vi "SLSC_Check Connection and Module.vi"(6 "Connect timeout (s)":dbl=4.0 format="%#_13g", 8 "error in (no error)":errorcluster, 10 "Supported Modules":T1[](array[typedef]), 11 "devices":refnum<k21>) -> (0 "error out":errorcluster, 3 "Device Found?":bool)   [LabVIEW 2015, in "SLSC CD Engine.lvlib"]
uses:
  SLSC CD API/SLSC CD Engine/SLSC CD Engine.lvlib
  SLSC CD API/SLSC CD Engine/SLSC Identification.ctl
  <vilib>/SLSC/Initialize Session with Devices.vi
  <vilib>/SLSC/Close Session.vi
  <vilib>/SLSC/SLSC.lvlib
  <resource>/objmgr/slsc.rc
  SLSC CD API/SLSC CD Shared/SLSC CD Shared.lvlib
panel:
  out "Supported Modules":T2(array[cluster]) {"Dev.ProductNumber" format="%.0x"; "Dev.VendorNumber" format="%.0x"}
  out "Dev.VendorNum":u32 format="%.0x"
  out "Dev.ProductNum":u32 format="%.0x"
  out "Dev.ProductName":string
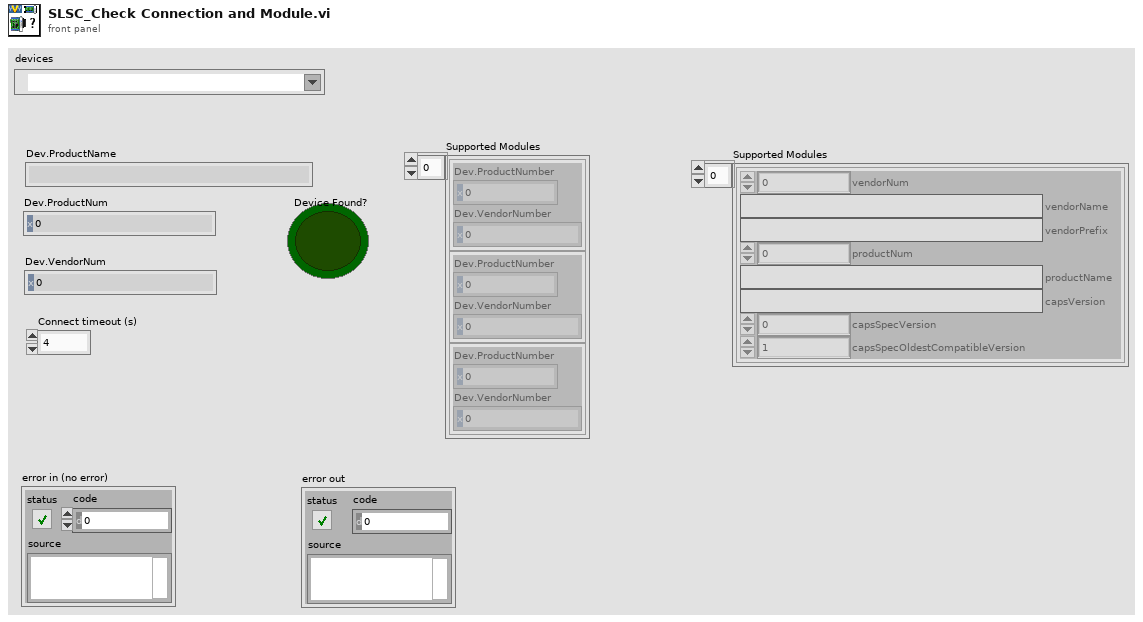
[diagram p1: front panel]
types:
  T1 = typedef "SLSC CD Shared.lvlib/SLSC Identification.ctl" = cluster{"vendorName":string, "productNum":u32, "capsVersion":string, "capsSpecVersion":u32, "productName":string, "vendorNum":u32, "vendorPrefix":string, "capsSpecOldestCompatibleVersion":u32}
  T2 = cluster{"Dev.ProductNumber":u32, "Dev.VendorNumber":u32}[]
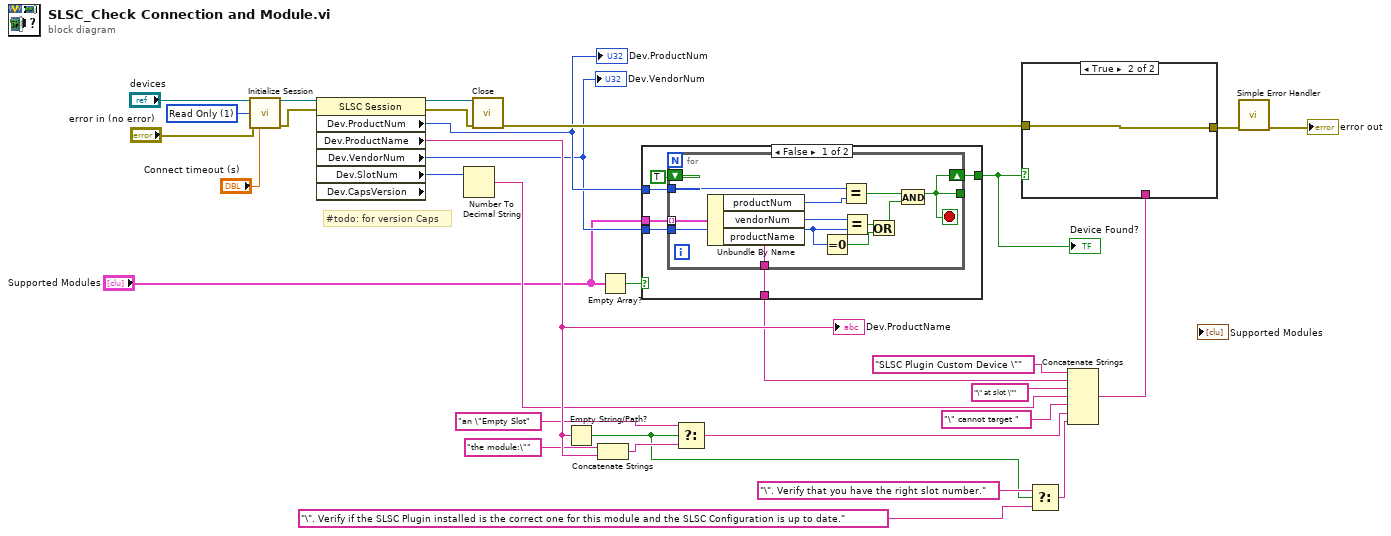
[diagram p0: block diagram]
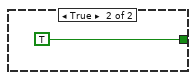
[diagram p2: hidden frame]
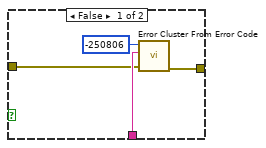
[diagram p3: hidden frame]
diagram:
  w8 = 1 items=["None"=0, "Read Only"=1, "Read/Write"=3] ("reservation access (Read/Write)")
  # "#todo: for version Caps"
  n1 = call-poly <vilib>:"Initialize Session.vi"("devices"="devices", "reservation access (Read/Write)"=w8, "error in (no error)"="error in (no error)", "connect timeout (60 sec)"="Connect timeout (s)") -> ("session out"=w13:refnum<k21>, "error out"=w12:errorcluster)  [unwired: 10 in]
  n2 = property class="SLSC Session" props=["Dev.ProductNum", "Dev.ProductName", "Dev.VendorNum", "Dev.SlotNum", "Dev.CapsVersion"](reference=w13, error in=w12) -> (reference out=w11:refnum<k21>, error out=w10:errorcluster, "Dev.ProductNum"=w18:u32, "Dev.ProductName"=w27:string, "Dev.VendorNum"=w17:u32, "Dev.SlotNum"=w7:u32)  [unwired: 1 out]
  "Dev.ProductName" <- w27
  "Dev.ProductNum" <- w18
  "Dev.VendorNum" <- w17
  n3 = Number To Decimal String(number=w7) -> (decimal integer string=w14:string)  [unwired: 1 in]
  n4 = call-poly <vilib>:"Close.vi"("session in"=w11, "error in (no error)"=w10) -> ("error out"=w32:errorcluster)  [unwired: 13 in]
  n5 = Empty String/Path?(string/path=w27) -> (empty?=w19:bool)
  n6 = Concatenate Strings("the module:\"" ("error message (\"\")"), w27) -> (w25:string)
  n7 = Empty Array?(array="Supported Modules") -> (empty?=w9:bool)
  n8 = case shown="False" w9 {
    tunnel: w18 -> [w37 _]
    tunnel: "Supported Modules" -> [w36 _]
    tunnel: w17 -> [w35 _]
    tunnel: [w34 TRUE] -> w1
    tunnel: [w33 _] -> w2
    frame False {
      n9 = for {
        tunnel: w37 -> [w49]
        tunnel: w36 -> [w40] mode=indexing
        tunnel: [w45] -> _
        shift-right: [w45] -> w34
        shift-left: TRUE ("x = y?") -> [_]
        tunnel: w35 -> [w44]
        tunnel: [w39] -> w33
        stop <- w45 stop-if-true
        n10 = Unbundle By Name(w40) -> ("productNum"=w47:u32, "vendorNum"=w46:u32, "productName"=w39:string)
        n11 = Equal To 0?(x=w44) -> (x = 0?=w42:bool)
        n12 = Equal?(x=w49, y=w47) -> (x = y?=w48:bool)
        n13 = Equal?(x=w46, y=w44) -> (x = y?=w43:bool)
        n14 = Or(x=w43, y=w42) -> (x .or. y?=w41:bool)
        n15 = And(x=w48, y=w41) -> (x .and. y?=w45:bool)
      }
    }
    frame True {
    }
  }
  "Device Found?" <- w1
  n16 = Select(t="an \"Empty Slot" ("error message (\"\")"), s=w19, f=w25) -> (s? t:f=w26:string)
  n17 = Select(t="\". Verify that you have the right slot number." ("string"), s=w19, f="\". Verify if the SLSC Plugin installed is the correct one for this module and the SLSC Configuration is up to date." ("string")) -> (s? t:f=w20:string)
  n18 = Concatenate Strings("SLSC Plugin Custom Device \"" ("error message (\"\")"), w2, "\" at slot \"" ("error message (\"\")"), w14, "\" cannot target " ("error message (\"\")"), w26, w20) -> (w31:string)
  n19 = case shown="True" w1 {
    tunnel: [w54 w55] -> w29
    tunnel: w32 -> [w51 w55]
    tunnel: w31 -> [w52 _]
    frame False {
      n20 = call <vilib>:"Error Cluster From Error Code.vi"("error in (no error)"=w51, "error message (\"\")"=w52, "error code (0)"=-250806) -> ("error out"=w54:errorcluster)  [unwired: 6 in]
    }
    frame True {
    }
  }
  n21 = call <vilib>:"Simple Error Handler.vi"("error in (no error)"=w29) -> ("error out"=→"error out":errorcluster)  [unwired: 4 in, 4 out]
